vi "DynamicEvent.vi"() -> ()   [LabVIEW 2010]
uses:
  <vilib>/Utility/miscctls.llb/LVPoint32TypeDef.ctl
panel:
  out "Mouse Up Coords":T1
  out "Mouse Down Coords":T1
  out "Mouse Move Coords":T1
  in  "stop":bool
  # "Drop any control on the panel in development sysytem and try to move its positon when running."
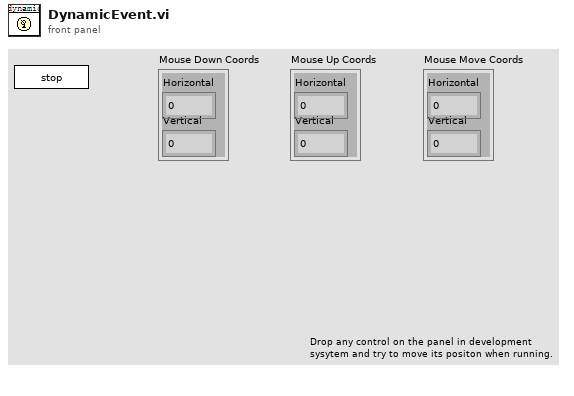
[diagram p1: front panel]
types:
  T1 = typedef "LVPoint32TypeDef.ctl" = cluster{"Horizontal":i32, "Vertical":i32}
  T2 = typedef "LVPositionTypeDef.ctl" = cluster{"Left":i32, "Top":i32}
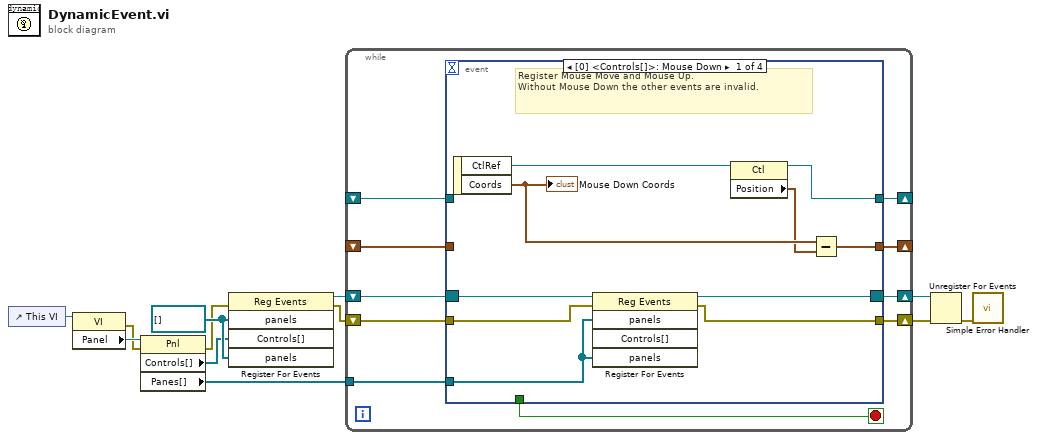
[diagram p0: block diagram]
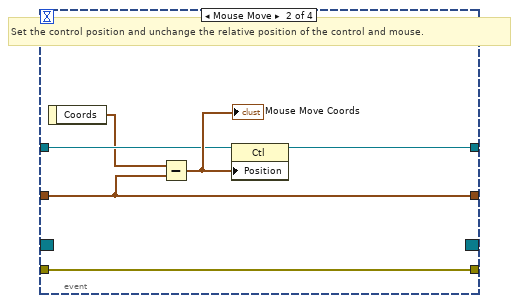
[diagram p2: hidden frame]
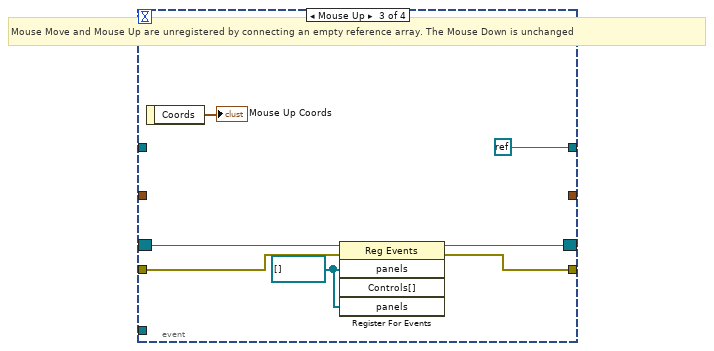
[diagram p3: hidden frame]
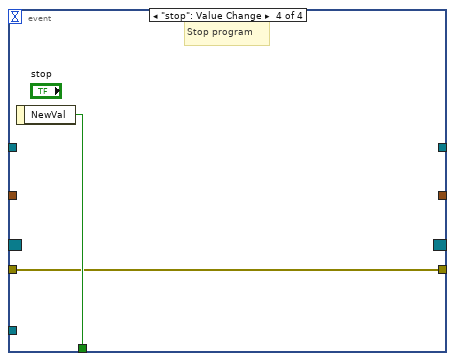
[diagram p4: hidden frame]
diagram:
  w8 = refnum<vi>[] [] ("panels")
  n1 = control-ref of="This VI"() -> (w11:refnum<vi>)
  n2 = property class="VI"(reference=w11) -> (error out=w5:errorcluster, "Panel"=w12:refnum<vi>)  [unwired: 1 in, 1 out]
  n3 = property class="Pnl"(reference=w12, error in=w5) -> (error out=w4:errorcluster, "Controls[]"=w7:refnum<vi>[], "Panes[]"=w6:refnum<vi>[])  [unwired: 1 out]
  n4 = register-events(error in=w4, w8, w7, w8) -> (reference out=w10:refnum<event-registration>, error out=w3:errorcluster)  [unwired: 1 in]
  n5 = while {
    shift-right: [w20] -> w9
    shift-left: w10 -> [w21]
    tunnel: w6 -> [w19]
    shift-right: [w18] -> _
    shift-left: _ -> [w17]
    shift-right: [w16] -> _
    shift-left: _ -> [w15]
    shift-right: [w13] -> w2
    shift-left: w3 -> [w14]
    stop <- w22 stop-if-true
    n6 = event shown="[0] <Controls[]>: Mouse Down" {
      selector: w21 -> [w31 _ w44 _]
      dyn-events: [w32 _ w42 _] -> w20
      timeout: _ -> [_ _ _ _]
      tunnel: [_ _ _ w47] -> w22
      tunnel: w19 -> [w30 _ _ _]
      tunnel: [w28 w34 refnum<k0> refnum _] -> w18
      tunnel: w17 -> [_ w37 _ _]
      tunnel: [w25 w35 _ _] -> w16
      tunnel: w15 -> [_ w35 _ _]
      tunnel: w14 -> [w24 w33 w40 w46]
      tunnel: [w23 w33 w39 w46] -> w13
      event Mouse Down {
        # "Register Mouse Move and Mouse Up.\nWithout Mouse Down the other events are invalid."
        n7 = event-data() -> ("CtlRef"=w29:refnum<vi>, "Coords"=w27:T1)  [unwired: 1 in]
        "Mouse Down Coords" <- w27
        n8 = register-events(reference=w31, error in=w24, w30, w30) -> (reference out=w32:refnum<event-registration>, error out=w23:errorcluster)  [unwired: 1 in]
        n9 = property class="Ctl"(reference=w29) -> (reference out=w28:refnum<vi>, "Position"=w26:T2)  [unwired: 1 in, 1 out]
        n10 = Subtract(x=w27, y=w26) -> (x-y=w25:T1)
      }
      event Mouse Move {
        # "Set the control position and unchange the relative position of the control and mouse."
        n11 = event-data() -> ("Coords"=w36:T1)  [unwired: 1 in]
        n12 = Subtract(x=w36, y=w35) -> (x-y=w38:T1)
        "Mouse Move Coords" <- w38
        n13 = property class="Ctl"(reference=w37, "Position"=w38) -> (reference out=w34:refnum<vi>)  [unwired: 1 in, 1 out]
      }
      event Mouse Up {
        w41 = refnum<vi>[] [] ("event source")
        # "Mouse Move and Mouse Up are unregistered by connecting an empty reference array. The Mouse Down is unchanged"
        n14 = event-data() -> ("Coords"=→"Mouse Up Coords":T1)  [unwired: 1 in]
        n15 = register-events(reference=w44, error in=w40, w41, w41) -> (reference out=w42:refnum<event-registration>, error out=w39:errorcluster)  [unwired: 1 in]
      }
      event "stop": Value Change {
        # "Stop program"
        n16 = event-data() -> ("NewVal"=w47:bool)  [unwired: 1 in]
      }
    }
  }
  n17 = Unregister For Events(event registration refnum=w9, error in=w2) -> (error out=w1:errorcluster)
  n18 = call <vilib>:"Simple Error Handler.vi"("error in (no error)"=w1) -> ()  [unwired: 4 in, 5 out]
